vi "in_bicubic poly coefs.vi"(11 "t":dbl) -> (3 "bicubic polynomial":dbl[](array[numeric]))   [LabVIEW 2018, in "NI_Gmath.lvlib"]
uses:
  NI_Gmath.lvlib
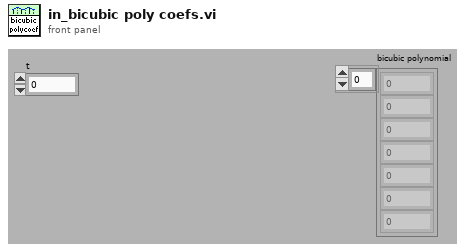
[diagram p1: front panel]
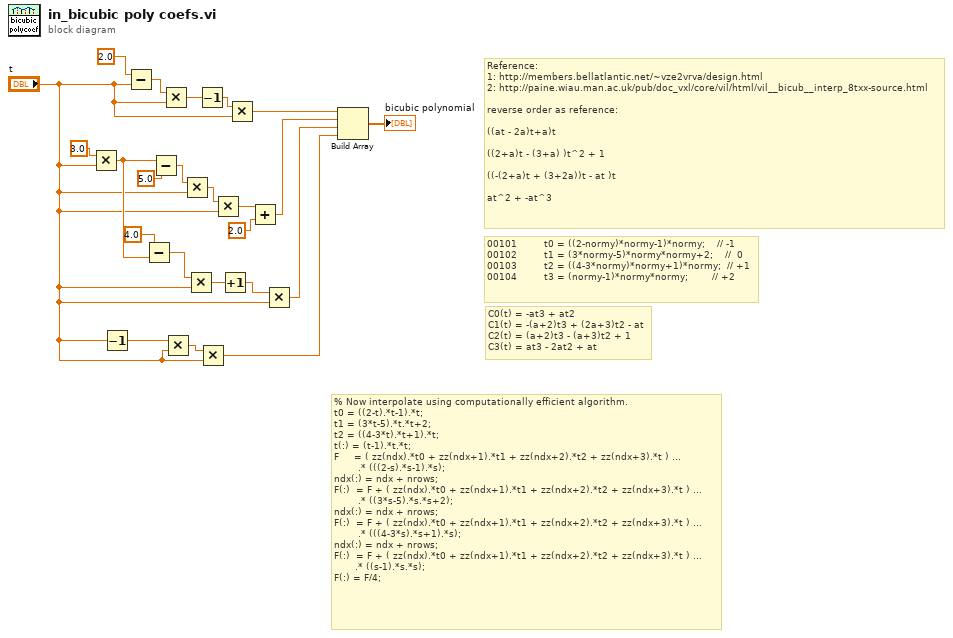
[diagram p0: block diagram]
diagram:
  # "% Now interpolate using computationally efficient algorithm.\nt0 = ((2-t).*t-1).*t;\nt1 = (3*t-5).*t.*t+2;\nt2 = ((4-3*t).*t+1).*t;\nt(:) = (t-1).*t.*t;\nF     = ( zz(ndx).*t0 + zz(ndx+1).*t1 + zz(ndx+2).*t2 + zz(ndx+3).*t ) ...\n        .* (((2-s).*s-1).*s);\nndx(:) = ndx + nrows;\nF(:)  = F + ( zz(ndx).*t0 + zz(ndx+1).*t1 + zz(ndx+2).*t2 + zz(ndx+3).*t ) ...\n        .* ((3*s-5).*s.*s+2);\nndx(:) = ndx + nrows;\nF(:)  = F + ( zz(ndx).*t0 + zz(ndx+1).*t1 + zz(ndx+2).*t2 + zz(ndx+3).*t ) ...\n        .* (((4-3*s).*s+1).*s);\nndx(:) = ndx + nrows;\nF(:)  = F + ( zz(ndx).*t0 + zz(ndx+1).*t1 + zz(ndx+2).*t2 + zz(ndx+3).*t ) ...\n       .* ((s-1).*s.*s);\nF(:) = F/4;"
  # "00101         t0 = ((2-normy)*normy-1)*normy;    // -1\n00102         t1 = (3*normy-5)*normy*normy+2;    //  0\n00103         t2 = ((4-3*normy)*normy+1)*normy;  // +1\n00104         t3 = (normy-1)*normy*normy;        // +2"
  # "Reference:\n1: http://members.bellatlantic.net/~vze2vrva/design.html \n2: http://paine.wiau.man.ac.uk/pub/doc_vxl/core/vil/html/vil__bicub__interp_8txx-source.html\n\nreverse order as reference:\n\n((at - 2a)t+a)t\n\n((2+a)t - (3+a) )t^2 + 1\n\n((-(2+a)t + (3+2a))t - at )t\n\nat^2 + -at^3"
  # "C0(t) = -at3 + at2 \nC1(t) = -(a+2)t3 + (2a+3)t2 - at \nC2(t) = (a+2)t3 - (a+3)t2 + 1 \nC3(t) = at3 - 2at2 + at"
  n1 = Multiply(x=3.0, y="t") -> (x*y=w10:dbl)
  n2 = Decrement(x="t") -> (x-1=w5:dbl)
  n3 = Subtract(x=2.0, y="t") -> (x-y=w22:dbl)
  n4 = Subtract(x=4.0, y=w10) -> (x-y=w9:dbl)
  n5 = Subtract(x=w10, y=5.0) -> (x-y=w16:dbl)
  n6 = Multiply(x=w22, y="t") -> (x*y=w21:dbl)
  n7 = Multiply(x=w5, y="t") -> (x*y=w3:dbl)
  n8 = Multiply(x=w16, y="t") -> (x*y=w15:dbl)
  n9 = Multiply(x=w9, y="t") -> (x*y=w8:dbl)
  n10 = Decrement(x=w21) -> (x-1=w20:dbl)
  n11 = Multiply(x=w3, y="t") -> (x*y=w2:dbl)
  n12 = Multiply(x=w15, y="t") -> (x*y=w14:dbl)
  n13 = Increment(x=w8) -> (x+1=w7:dbl)
  n14 = Multiply(x=w20, y="t") -> (x*y=w19:dbl)
  n15 = Add(x=w14, y=2.0) -> (x+y=w12:dbl)
  n16 = Multiply(x=w7, y="t") -> (x*y=w6:dbl)
  n17 = Build Array(w19, w12, w6, w2) -> (→"bicubic polynomial":dbl[])
